vi "svfa_Locate Three Fingers (complex).vi"(3 "criterion":T1={"Single/Multiple"=enum."Multiple Peaks", "Threshold"=0.0, "advanced search"={"approximate frequencies"=[], "advanced span [Hz]"=5.0}} {"advanced search"."advanced span [Hz]" format="%0.2p"; "Threshold" format="%.2f"}, 5 "complex spectrum":T8={"complex spectrum response"={"f0"=0.0, "df"=1.0, "complex spectrum"=[]}, "spectrum info"={"channel name"="", "description"="", "x-axis units"=0, "spectral info"={"spectrum type"=enum."Power [Magnitude^2]", "linear/dB"=enum."linear", "window"=0, "window size"=0, "FFT size"=0}, "engineering units"=0, "custom label"="", "dB reference [EU]"=0.0, "peak units"=enum."rms", "weighting filter"=0, "spectral density?"=FALSE, "unit label"="", "spectrum skewed?"=FALSE, "complimentary spectrum units"=enum."none"}} {"spectrum info"."x-axis units" items=["Time (s)"=0, "Frequency-CB (Hz)"=1, "Frequency-CPB (Hz)"=1248, "Frequency-Arbitrary (Hz)"=2357, "Quefrency (s)"=2, "Revolutions (rev)"=3, "Order"=4, "Speed (RPM)"=11, "Speed (rad/s)"=21, "Index"=65535]; "spectrum info"."weighting filter" items=["Linear", "A-weighting", "B-weighting", "C-weighting", "ITU-R 468-4", "Dolby", "CCITT", "C-message", "Wb", "Wc", "Wd", "We", "Wf", "Wh", "Wj", "Wk", "Wm", "AES17 20 kHz lowpass", "AES17 40 kHz lowpass", "AES17 20 kHz highpass", "AES17 40 kHz highpass"]; "spectrum info"."dB reference [EU]" format="%.2f"; "spectrum info"."engineering units" items=["custom..."=0, "V"=1, "A"=21, "C"=30, "pC"=31, "s"=32, "-"=29, "Pa"=2, "N"=20, "g"=3, "m/s^2"=4, "m/s"=5, "m"=6, "mm/s"=12, "mm"=13, "micron/s"=14, "micron"=15, "in/s^2"=7, "in/s"=8, "in"=9, "mil/s"=10, "mil"=11, "rad/s^2"=16, "rad/s"=17, "rad"=18, "deg/s^2"=26, "deg/s"=27, "deg"=28, "RPM"=22, "cycle/s^2"=23, "Hz"=24, "cycle"=25, "strain"=19]; "spectrum info"."spectral info"."window" items=["None "=0, "Hanning"=1, "Hamming"=2, "Blackman-Harris"=3, "Exact Blackman"=4, "Blackman"=5, "Flat Top"=6, "4 Term B-Harris "=7, "7 Term B-Harris"=8, "Low Sidelobe"=9, "Force - Exponential"=10, "Gaussian"=62]; "complex spectrum response"."complex spectrum" format="%.2f"; "complex spectrum response"."df" format="%.2f"; "complex spectrum response"."f0" format="%.2f"}) -> (0 "number of tones":i32, 1 "three fingers (frequency normorlized)":cluster{"f0":dbl, "df":dbl, "spectrum":cdb[]}[](array[cluster]) {"spectrum" format="%.2f"; "df" format="%.2f"; "f0" format="%.2f"}, 2 "exact normalized frequencies?":dbl[](array[numeric]))   [LabVIEW 2017]
uses:
  <vilib>/addons/_NISVFA/_Shared subVIs/Controls/svc_Spectrum Info.ctl
  <vilib>/addons/_NISVFA/_Shared subVIs/Controls/svc_X-Axis Units.ctl
  <vilib>/addons/_NISVFA/_Shared subVIs/Controls/svc_Spectrum Type.ctl
  <vilib>/addons/_NISVFA/_Shared subVIs/Controls/svc_Engineering Units Text Ring.ctl
  <vilib>/addons/_NISVFA/_Shared subVIs/Controls/svc_Weighting Filter Text Ring.ctl
  <vilib>/addons/_NISVFA/_Shared subVIs/Controls/svc_Complimentary Spectrum Units.ctl
  <vilib>/Analysis/_algsub.llb/Complex Vector Norm.vi
  <vilib>/addons/_NISVFA/_Spectrum Processing/SVFA Get Spectrum Subset (Complex) (1 Ch).vi
  <vilib>/Analysis/NI_AALPro.lvlib
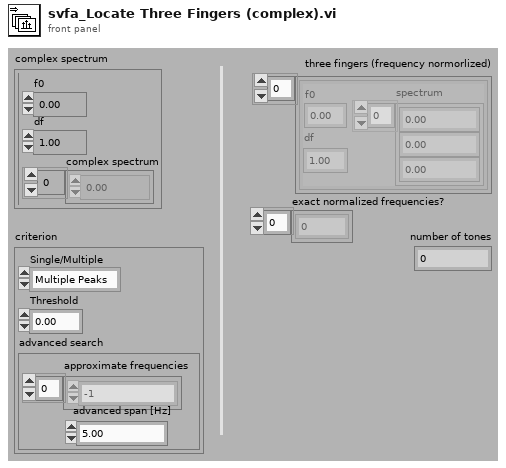
[diagram p1: front panel]
types:
  T1 = cluster{"Single/Multiple":enum16{"Multiple Peaks", "Single Max Peak"}, "Threshold":dbl, "advanced search":cluster{"approximate frequencies":dbl[], "advanced span [Hz]":dbl}}
  T2 = typedef "svc_Spectrum Info.ctl" = cluster{"channel name":string, "description":string, "x-axis units":T3, "spectral info":cluster{"spectrum type":T4, "linear/dB":enum16{"linear", "dB"}, "window":u16, "window size":i32, "FFT size":i32}, "engineering units":T5, "custom label":string, "dB reference [EU]":dbl, "peak units":enum16{"rms", "peak", "peak-peak"}, "weighting filter":T6, "spectral density?":bool, "unit label":string, "spectrum skewed?":bool, "complimentary spectrum units":T7}
  T3 = typedef "svc_X-Axis Units.ctl" = u16
  T4 = typedef "svc_Spectrum Type.ctl" = enum16{"FFT Spectrum [complex]", "Amplitude [Magnitude]", "Power [Magnitude^2]", "Cross Spectrum [complex]", "Frequency Response [Complex]"}
  T5 = typedef "svc_Engineering Units Text Ring.ctl" = u16
  T6 = typedef "svc_Weighting Filter Text Ring.ctl" = u16
  T7 = typedef "svc_Complimentary Spectrum Units.ctl" = enum16{"none", "radians", "degrees", "cycles", "imaginary"}
  T8 = cluster{"complex spectrum response":cluster{"f0":dbl, "df":dbl, "complex spectrum":cdb[]}, "spectrum info":T2}
  T9 = cluster{"start frequency":dbl, "stop frequency":dbl}
  T10 = cluster{"complex spectrum subset":cluster{"x0":dbl, "dx":dbl, "complex array":cdb[]}, "spectrum info":T2}
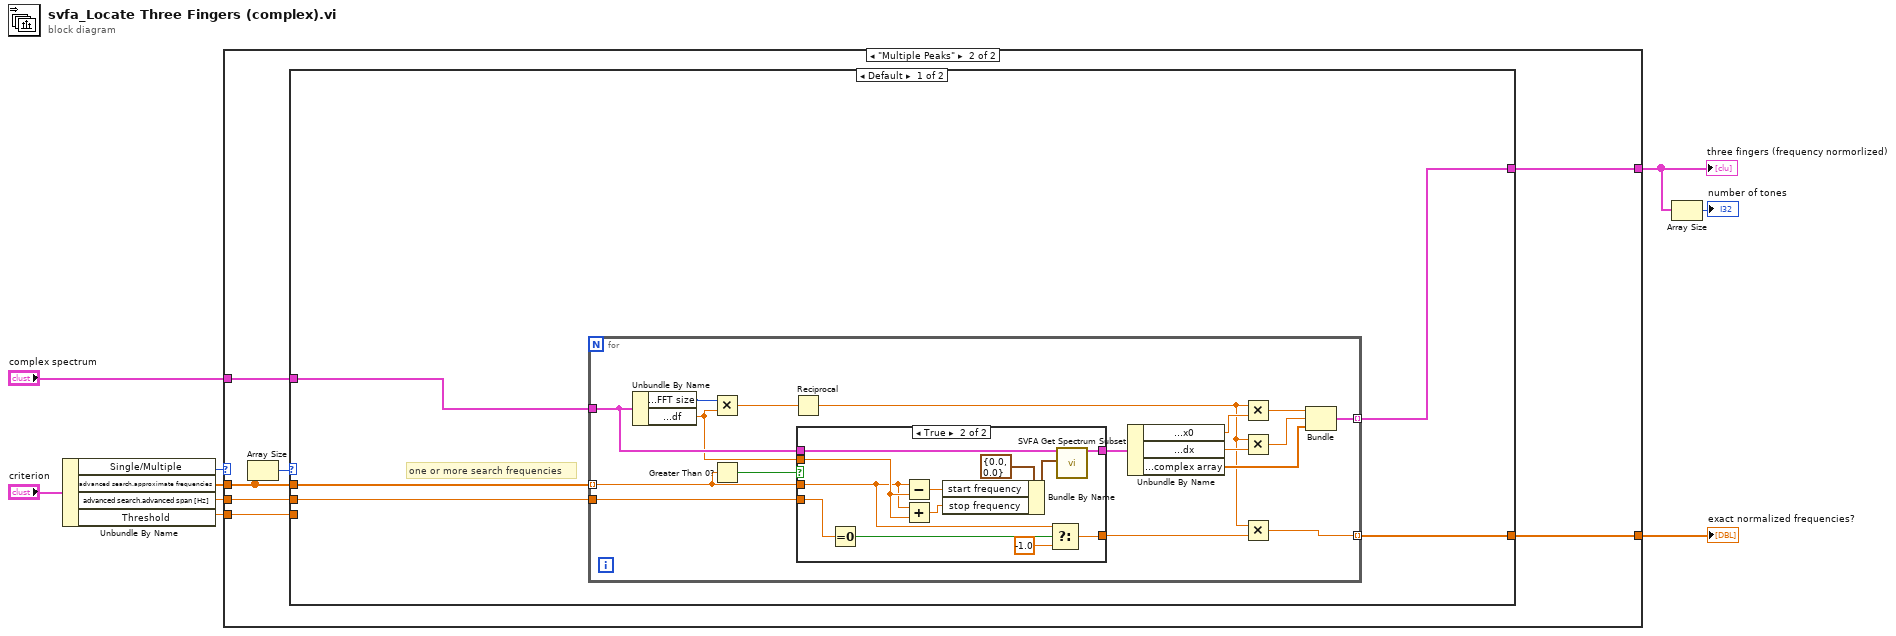
[diagram p0: block diagram]
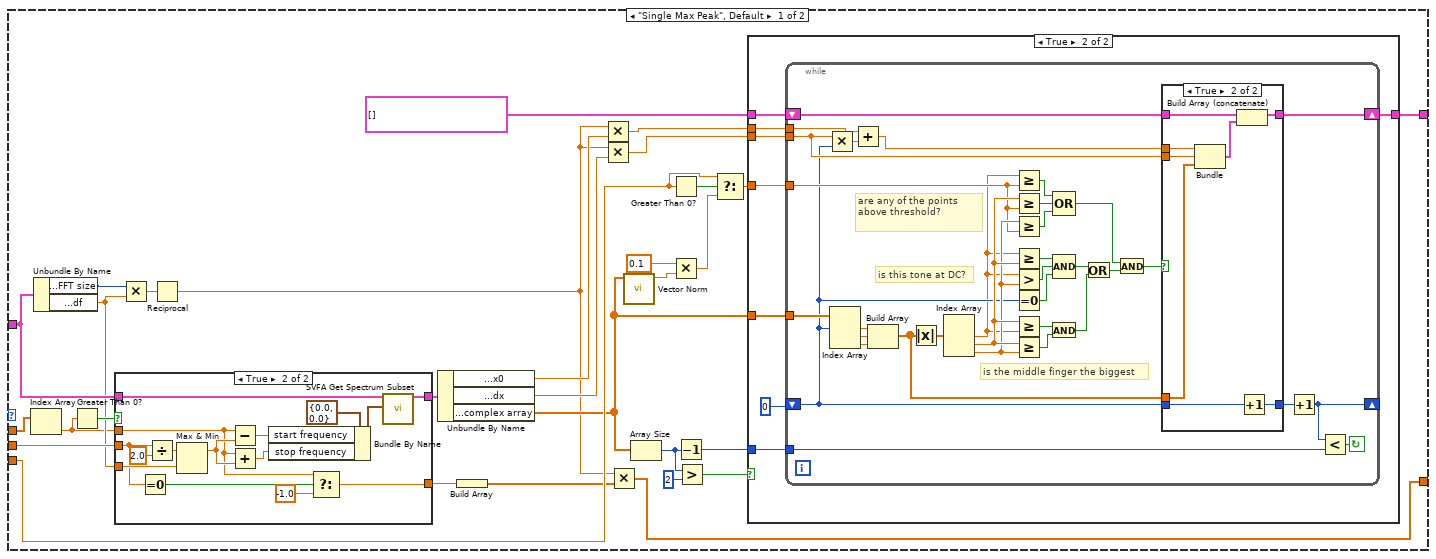
[diagram p2: hidden frame]
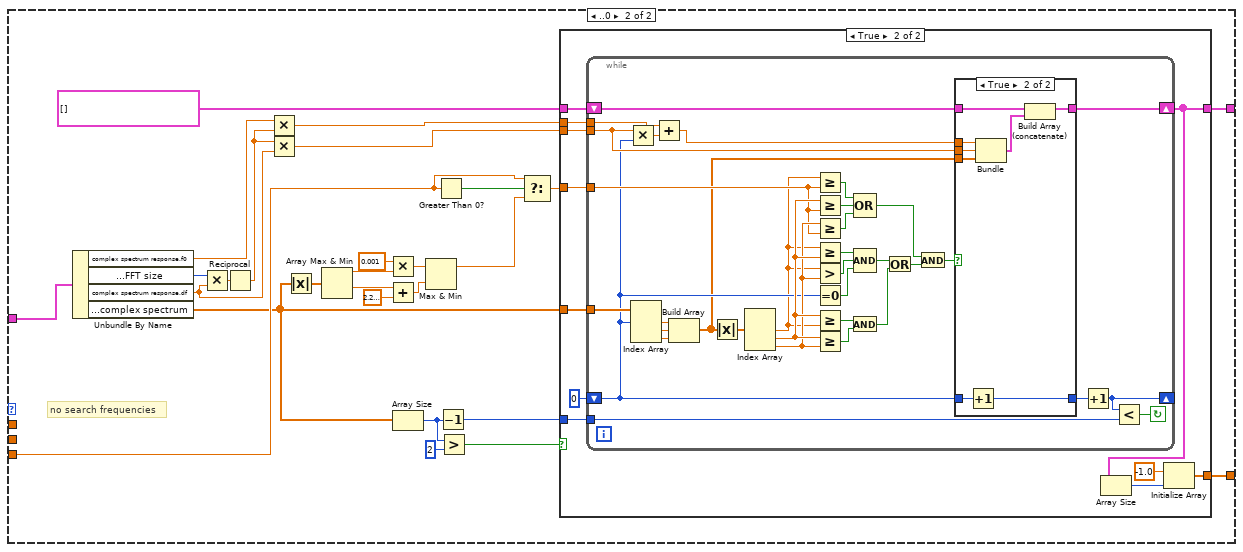
[diagram p7: hidden frame]
diagram:
  n1 = Unbundle By Name("criterion") -> ("Single/Multiple"=w3:enum16{"Multiple Peaks", "Single Max Peak"}, "advanced search.approximate frequencies"=w2:dbl[], "advanced search.advanced span [Hz]"=w7:dbl, "Threshold"=w4:dbl)
  n2 = case shown="\"Multiple Peaks\"" w3 {
    tunnel: [w37 w114] -> w9
    tunnel: w7 -> [w33 w116]
    tunnel: "complex spectrum" -> [w31 w115]
    tunnel: w2 -> [w22 w111]
    tunnel: w4 -> [w15 w113]
    tunnel: [w10 w110] -> w1
    frame "Single Max Peak", Default {
      n3 = Index Array(array=w22) -> (element=w21:dbl)  [unwired: 1 in]
      n4 = Unbundle By Name(w31) -> ("spectrum info.spectral info.FFT size"=w34:i32, "complex spectrum response.df"=w28:dbl)
      n5 = Greater Than 0?(x=w21) -> (x > 0?=w30:bool)
      n6 = case shown="True" w30 {
        tunnel: w33 -> [_ w46]
        tunnel: w21 -> [w40 w44]
        tunnel: w31 -> [w41 w49]
        tunnel: w28 -> [_ w53]
        tunnel: [w41 w48] -> w25
        tunnel: [w40 w42] -> w13
        frame False {
        }
        frame True {
          n7 = Equal To 0?(x=w46) -> (x = 0?=w45:bool)
          n8 = Divide(x=w46, y=2.0) -> (x/y=w50:dbl)
          n9 = Max & Min(x=w50, y=w53) -> (max(x,y)=w52:dbl)  [unwired: 1 out]
          n10 = Subtract(x=w44, y=w52) -> (x-y=w56:dbl)
          n11 = Add(x=w44, y=w52) -> (x+y=w55:dbl)
          n12 = Bundle By Name(cluster=T9 {"start frequency"=0.0, "stop frequency"=0.0} ("frequency range"), "start frequency"=w56, "stop frequency"=w55) -> (w54:T9)
          n13 = Select(t=w44, s=w45, f=-1.0) -> (s? t:f=w42:dbl)
          n14 = call-poly <vilib>:"SVFA Get Spectrum Subset.vi"("complex spectrum"=w49, "range"=w54) -> ("complex spectrum subset"=w48:T10)  [unwired: 14 in, 3 out]
        }
      }
      n15 = Multiply(x=w34, y=w28) -> (x*y=w32:dbl)
      n16 = Reciprocal(x=w32) -> (1/x=w12:dbl)
      n17 = Unbundle By Name(w25) -> ("complex spectrum subset.x0"=w29:dbl, "complex spectrum subset.dx"=w27:dbl, "complex spectrum subset.complex array"=w14:cdb[])
      n18 = Build Array(w13) -> (w11:dbl[])
      n19 = Multiply(x=w12, y=w29) -> (x*y=w36:dbl)
      n20 = Multiply(x=w12, y=w27) -> (x*y=w35:dbl)
      n21 = Multiply(x=w12, y=w11) -> (x*y=w10:dbl[])
      n22 = call-poly <vilib>:"Vector Norm.vi"("Input Vector"=w14) -> ("norm"=w20:dbl)  [unwired: 9 in, 1 out]
      n23 = Array Size(array=w14) -> (size(s)=w23:i32)
      n24 = Greater Than 0?(x=w15) -> (x > 0?=w19:bool)
      n25 = Multiply(x=0.1, y=w20) -> (x*y=w16:dbl)
      n26 = Decrement(x=w23) -> (x-1=w24:i32)
      n27 = Greater?(x=w23, y=2) -> (0:w39:bool)
      n28 = Select(t=w15, s=w19, f=w16) -> (s? t:f=w17:dbl)
      n29 = case shown="True" w39 {
        tunnel: w36 -> [_ w65]
        tunnel: w35 -> [_ w64]
        tunnel: [w57 w63] -> w37
        tunnel: w14 -> [_ w59]
        tunnel: cluster{"f0":dbl, "df":dbl, "spectrum":cdb[]}[] [] ("three fingers") -> [w57 w62]
        tunnel: w24 -> [_ w60]
        tunnel: w17 -> [_ w58]
        frame False {
        }
        frame True {
          n30 = while {
            tunnel: w60 -> [w93]
            tunnel: w64 -> [w75]
            tunnel: w65 -> [w76]
            tunnel: w59 -> [w77]
            shift-left: w62 -> [w97]
            shift-right: [w96] -> w63
            tunnel: w58 -> [w88]
            shift-left: 0 -> [w74]
            shift-right: [w94] -> _
            stop <- w95 continue-if-true
            # "is the middle finger the biggest"
            # "is this tone at DC?"
            # "are any of the points above threshold?"
            n31 = Multiply(x=w75, y=w74) -> (x*y=w67:dbl)
            n32 = Index Array(array=w77, index #1=w74) -> (element #1=w71:cdb, element #2=w72:cdb, element #3=w70:cdb)  [unwired: 2 in]
            n33 = Add(x=w76, y=w67) -> (x+y=w73:dbl)
            n34 = Build Array(w71, w72, w70) -> (w66:cdb[])
            n35 = Absolute Value(x=w66) -> (abs(x)=w68:dbl[])
            n36 = Index Array(array=w68) -> (element #1=w69:dbl, element #2=w92:dbl, element #3=w91:dbl)  [unwired: 3 in]
            n37 = Greater Or Equal?(x=w69, y=w88) -> (x >= y?=w90:bool)
            n38 = Greater Or Equal?(x=w92, y=w88) -> (x >= y?=w99:bool)
            n39 = Greater Or Equal?(x=w91, y=w88) -> (x >= y?=w89:bool)
            n40 = Greater Or Equal?(x=w69, y=w92) -> (x >= y?=w86:bool)
            n41 = Greater?(x=w69, y=w91) -> (0:w85:bool)
            n42 = Equal To 0?(x=w74) -> (x = 0?=w84:bool)
            n43 = Greater Or Equal?(x=w92, y=w69) -> (x >= y?=w87:bool)
            n44 = Greater Or Equal?(x=w92, y=w91) -> (x >= y?=w82:bool)
            n45 = And(x=w87, y=w82) -> (x .and. y?=w81:bool)
            n46 = Compound Arithmetic op=OR(w90, w99, w89) -> (w79:bool)
            n47 = Compound Arithmetic op=AND(w86, w85, w84) -> (w83:bool)
            n48 = Or(x=w83, y=w81) -> (x .or. y?=w80:bool)
            n49 = And(x=w79, y=w80) -> (x .and. y?=w78:bool)
            n50 = case shown="True" w78 {
              tunnel: w74 -> [w101 w108]
              tunnel: [w101 w109] -> w98
              tunnel: w97 -> [w100 w106]
              tunnel: w75 -> [_ w107]
              tunnel: [w100 w104] -> w96
              tunnel: w66 -> [_ w103]
              tunnel: w73 -> [_ w102]
              frame False {
              }
              frame True {
                n51 = Bundle(w102, w107, w103) -> (w105:cluster{dbl, dbl, cdb[]})  [unwired: 1 in]
                n52 = Build Array (concatenate)(w106, w105) -> (w104:cluster{"f0":dbl, "df":dbl, "spectrum":cdb[]}[])
                n53 = Increment(x=w108) -> (x+1=w109:i32)
              }
            }
            n54 = Increment(x=w98) -> (x+1=w94:i32)
            n55 = Less?(x=w94, y=w93) -> (x < y?=w95:bool)
          }
        }
      }
    }
    frame "Multiple Peaks" {
      n56 = Array Size(array=w111) -> (size(s)=w112:i32)
      n57 = case shown="Default" w112 {
        tunnel: w116 -> [w121 _]
        tunnel: w115 -> [w120 w171]
        tunnel: w111 -> [w119 _]
        tunnel: [w118 w163] -> w114
        tunnel: w113 -> [_ w164]
        tunnel: [w117 w153] -> w110
        frame Default {
          # "one or more search frequencies"
          n58 = for {
            tunnel: w121 -> [w137]
            tunnel: w120 -> [w135]
            tunnel: w119 -> [w126] mode=indexing
            tunnel: [w125] -> w118 mode=indexing
            tunnel: [w122] -> w117 mode=indexing
            n59 = Unbundle By Name(w135) -> ("spectrum info.spectral info.FFT size"=w138:i32, "complex spectrum response.df"=w132:dbl)
            n60 = Multiply(x=w138, y=w132) -> (x*y=w136:dbl)
            n61 = Greater Than 0?(x=w126) -> (x > 0?=w134:bool)
            n62 = Reciprocal(x=w136) -> (1/x=w124:dbl)
            n63 = case shown="True" w134 {
              tunnel: w137 -> [_ w145]
              tunnel: w126 -> [w139 w143]
              tunnel: w135 -> [w140 w149]
              tunnel: w132 -> [_ w146]
              tunnel: [w140 w148] -> w130
              tunnel: [w139 w141] -> w123
              frame False {
              }
              frame True {
                n64 = Equal To 0?(x=w145) -> (x = 0?=w144:bool)
                n65 = Subtract(x=w143, y=w146) -> (x-y=w152:dbl)
                n66 = Add(x=w143, y=w146) -> (x+y=w151:dbl)
                n67 = Bundle By Name(cluster=T9 {"start frequency"=0.0, "stop frequency"=0.0} ("frequency range"), "start frequency"=w152, "stop frequency"=w151) -> (w150:T9)
                n68 = Select(t=w143, s=w144, f=-1.0) -> (s? t:f=w141:dbl)
                n69 = call-poly <vilib>:"SVFA Get Spectrum Subset.vi"("complex spectrum"=w149, "range"=w150) -> ("complex spectrum subset"=w148:T10)  [unwired: 14 in, 3 out]
              }
            }
            n70 = Unbundle By Name(w130) -> ("complex spectrum subset.x0"=w133:dbl, "complex spectrum subset.dx"=w131:dbl, "complex spectrum subset.complex array"=w129:cdb[])
            n71 = Multiply(x=w124, y=w133) -> (x*y=w128:dbl)
            n72 = Multiply(x=w124, y=w131) -> (x*y=w127:dbl)
            n73 = Multiply(x=w124, y=w123) -> (x*y=w122:dbl)
            n74 = Bundle(w128, w127, "complex array"=w129) -> (w125:cluster{dbl, dbl, "complex array":cdb[]})  [unwired: 1 in]
          }
        }
        frame ..0 {
          # "no search frequencies"
          n75 = Unbundle By Name(w171) -> ("complex spectrum response.f0"=w162:dbl, "spectrum info.spectral info.FFT size"=w174:i32, "complex spectrum response.df"=w161:dbl, "complex spectrum response.complex spectrum"=w160:cdb[])
          n76 = Multiply(x=w174, y=w161) -> (x*y=w173:dbl)
          n77 = Reciprocal(x=w173) -> (1/x=w175:dbl)
          n78 = Multiply(x=w162, y=w175) -> (x*y=w177:dbl)
          n79 = Multiply(x=w175, y=w161) -> (x*y=w176:dbl)
          n80 = Absolute Value(x=w160) -> (abs(x)=w159:dbl[])
          n81 = Array Max & Min(array=w159) -> (max value=w168:dbl, min value=w158:dbl)  [unwired: 2 out]
          n82 = Multiply(x=0.001, y=w168) -> (x*y=w156:dbl)
          n83 = Add(x=w158, y=2.220446049250313e-16 ("x")) -> (x+y=w155:dbl)
          n84 = Array Size(array=w160) -> (size(s)=w169:i32)
          n85 = Max & Min(x=w156, y=w155) -> (max(x,y)=w154:dbl)  [unwired: 1 out]
          n86 = Greater Than 0?(x=w164) -> (x > 0?=w167:bool)
          n87 = Decrement(x=w169) -> (x-1=w170:i32)
          n88 = Greater?(x=w169, y=2) -> (0:w179:bool)
          n89 = Select(t=w164, s=w167, f=w154) -> (s? t:f=w165:dbl)
          n90 = case shown="True" w179 {
            tunnel: w177 -> [_ w191]
            tunnel: w176 -> [_ w190]
            tunnel: [w180 w184] -> w163
            tunnel: w160 -> [_ w186]
            tunnel: cluster{"f0":dbl, "df":dbl, "spectrum":cdb[]}[] [] ("three fingers") -> [w180 w189]
            tunnel: w170 -> [_ w187]
            tunnel: w165 -> [_ w185]
            tunnel: [_ w181] -> w153
            frame False {
            }
            frame True {
              n91 = while {
                tunnel: w187 -> [w219]
                tunnel: w190 -> [w201]
                tunnel: w191 -> [w202]
                tunnel: w186 -> [w203]
                shift-left: w189 -> [w223]
                shift-right: [w222] -> w184
                tunnel: w185 -> [w214]
                shift-left: 0 -> [w200]
                shift-right: [w220] -> _
                stop <- w221 continue-if-true
                n92 = Multiply(x=w201, y=w200) -> (x*y=w192:dbl)
                n93 = Index Array(array=w203, index #1=w200) -> (element #1=w197:cdb, element #2=w198:cdb, element #3=w196:cdb)  [unwired: 2 in]
                n94 = Add(x=w202, y=w192) -> (x+y=w199:dbl)
                n95 = Build Array(w197, w198, w196) -> (w195:cdb[])
                n96 = Absolute Value(x=w195) -> (abs(x)=w193:dbl[])
                n97 = Index Array(array=w193) -> (element #1=w194:dbl, element #2=w218:dbl, element #3=w217:dbl)  [unwired: 3 in]
                n98 = Greater Or Equal?(x=w194, y=w214) -> (x >= y?=w216:bool)
                n99 = Greater Or Equal?(x=w218, y=w214) -> (x >= y?=w225:bool)
                n100 = Greater Or Equal?(x=w217, y=w214) -> (x >= y?=w215:bool)
                n101 = Greater Or Equal?(x=w194, y=w218) -> (x >= y?=w212:bool)
                n102 = Greater?(x=w194, y=w217) -> (0:w211:bool)
                n103 = Equal To 0?(x=w200) -> (x = 0?=w210:bool)
                n104 = Greater Or Equal?(x=w218, y=w194) -> (x >= y?=w213:bool)
                n105 = Greater Or Equal?(x=w218, y=w217) -> (x >= y?=w208:bool)
                n106 = And(x=w213, y=w208) -> (x .and. y?=w207:bool)
                n107 = Compound Arithmetic op=OR(w216, w225, w215) -> (w205:bool)
                n108 = Compound Arithmetic op=AND(w212, w211, w210) -> (w209:bool)
                n109 = Or(x=w209, y=w207) -> (x .or. y?=w206:bool)
                n110 = And(x=w205, y=w206) -> (x .and. y?=w204:bool)
                n111 = case shown="True" w204 {
                  tunnel: w200 -> [w227 w234]
                  tunnel: [w227 w235] -> w224
                  tunnel: w223 -> [w226 w232]
                  tunnel: w201 -> [_ w233]
                  tunnel: [w226 w230] -> w222
                  tunnel: w195 -> [_ w229]
                  tunnel: w199 -> [_ w228]
                  frame False {
                  }
                  frame True {
                    n112 = Increment(x=w234) -> (x+1=w235:i32)
                    n113 = Bundle(w228, w233, w229) -> (w231:cluster{dbl, dbl, cdb[]})  [unwired: 1 in]
                    n114 = Build Array (concatenate)(w232, w231) -> (w230:cluster{"f0":dbl, "df":dbl, "spectrum":cdb[]}[])
                  }
                }
                n115 = Increment(x=w224) -> (x+1=w220:i32)
                n116 = Less?(x=w220, y=w219) -> (x < y?=w221:bool)
              }
              n117 = Array Size(array=w184) -> (size(s)=w183:i32)
              n118 = Initialize Array(-1.0 ("element"), w183) -> (w181:dbl[])
            }
          }
        }
      }
    }
  }
  "three fingers (frequency normorlized)" <- w9
  "exact normalized frequencies?" <- w1
  n119 = Array Size(array=w9) -> (size(s)=→"number of tones":i32)
